vi "Cache_Hierarchy Global_Load All.vi"(8 "error in (no error)":errorcluster) -> (0 "error out":errorcluster, 1 "All Success?":bool, 3 "Hierarchy Map":map{string, string[]}(c390))   [LabVIEW 2019, in "ClassLoader.lvlib"]
doc: "Return paths to the ini cache files for all loaded PPLs."
uses:
  ClassLoader.lvlib
  Cache_Hierarchy Global.vi
  <vilib>/Utility/config.llb/NI_LVConfig.lvlib
  Ctl/Ctl_Hierarchy Cluster.ctl
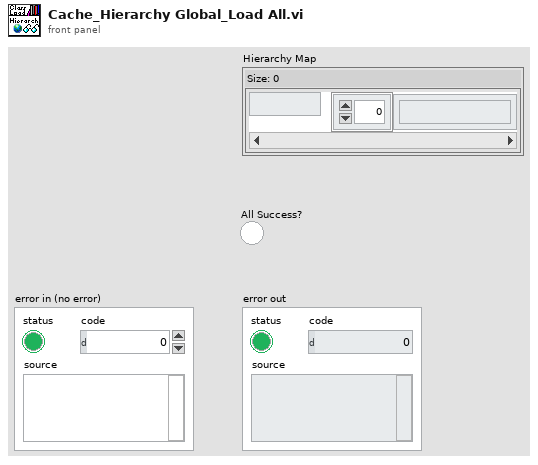
[diagram p1: front panel]
types:
  T1 = typedef "ClassLoader.lvlib/Ctl_Hierarchy Cluster.ctl" = cluster{"Hierarchy":string[]}
  T2 = typedef "NI_LVConfig.lvlib/Config Data RefNum.ctl" = refnum<k1>
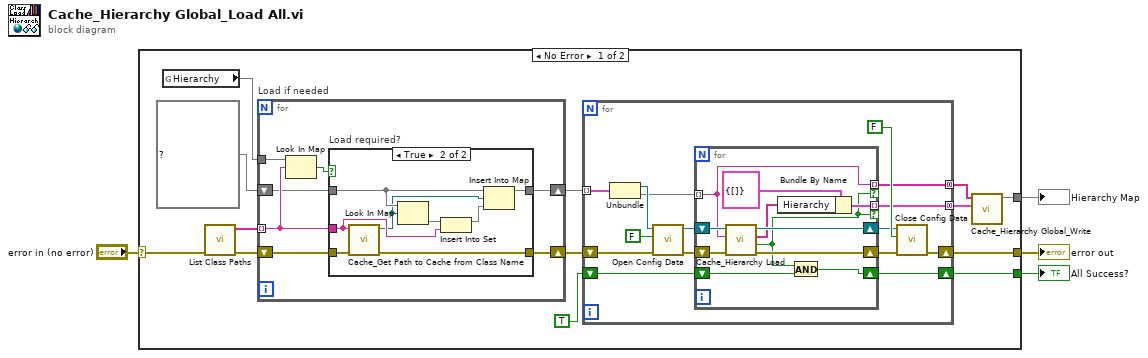
[diagram p0: block diagram]
diagram:
  n1 = case shown="No Error" "error in (no error)" {
    selector: "error in (no error)" -> [w17 w61]
    tunnel: [w10 w61] -> w3
    tunnel: [w7 _] -> w2
    tunnel: [w5 _] -> w1
    frame No Error {
      n2 = global read "Cache_Hierarchy Global.vi" "Hierarchy"() -> (w12:map{string, string[]})
      n3 = call "List Class Paths.vi"("error in (no error)"=w17) -> ("error out"=w13:errorcluster, "Class Names"=w16:string[])  [unwired: 8 in, 1 out]
      n4 = for "Load if needed" {
        tunnel: w16 -> [w48] mode=indexing
        tunnel: w12 -> [w49]
        shift-right: [w46] -> w11
        shift-left: map{path, set{string}} {} ("map") -> [w47]
        shift-right: [w45] -> w14
        shift-left: w13 -> [w44]
        n5 = Look In Map(map=w49, key=w48) -> (key not found?=w50:bool)  [unwired: 1 in, 1 out]
        n6 = case "Load required?" shown="True" w50 {
          tunnel: w48 -> [_ w59]
          tunnel: w47 -> [w52 w58]
          tunnel: [w52 w57] -> w46
          tunnel: [w51 w53] -> w45
          tunnel: w44 -> [w51 w54]
          frame False {
          }
          frame True {
            n7 = call "Cache_Get Path to Cache from Class Name.vi"("error in (no error)"=w54, "Class Name"=w59) -> ("error out"=w53:errorcluster, "Cache Path"=w56:path)  [unwired: 7 in, 1 out]
            n8 = Look In Map(map=w58, key=w56) -> (value=w60:set{string})  [unwired: 1 in, 1 out]
            n9 = Insert Into Set(10:w59, 11:w60) -> (3:w55:set{string})  [unwired: 1 out]
            n10 = Insert Into Map(map in=w58, key=w56, value=w55) -> (map out=w57:map{path, set{string}})  [unwired: 2 out]
          }
        }
      }
      n11 = for {
        tunnel: w11 -> [w32] mode=indexing
        shift-right: [w22] -> w10
        shift-left: w14 -> [w29]
        tunnel: [w21] -> w8 mode=concatenating
        tunnel: [w20] -> w9 mode=concatenating
        shift-right: [w18] -> w5
        shift-left: TRUE -> [w19]
        n12 = Unbundle(w32) -> ("Cache Path"=w30:path, "set"=w26:set{string})
        n13 = call <vilib>:"Open Config Data.vi"("error in (no error)"=w29, "create file if necessary (T)"=FALSE, "configuration file path"=w30) -> ("error out"=w24:errorcluster, "refnum"=w27:T2)  [unwired: 6 in, 1 out]
        n14 = for {
          shift-right: [w42] -> w25
          shift-left: w27 -> [w43]
          tunnel: w26 -> [w36] mode=indexing
          shift-right: [w40] -> w23
          shift-left: w24 -> [w41]
          tunnel: [w37] -> w21 mode=indexing if=w33
          tunnel: [w36] -> w20 mode=indexing if=w33
          shift-right: [w34] -> w18
          shift-left: w19 -> [w35]
          n15 = call "Cache_Hierarchy Load.vi"("error in (no error)"=w41, "Class Name"=w36, "Refnum in"=w43) -> ("error out"=w40:errorcluster, "Success?"=w33:bool, "Hierarchy"=w38:string[], "Refnum out"=w42:T2)  [unwired: 5 in]
          n16 = Bundle By Name(cluster=T1 {"Hierarchy"=[]} ("Hierarchy Cluster"), "Hierarchy"=w38) -> (w37:T1)
          n17 = And(x=w33, y=w35) -> (x .and. y?=w34:bool)
        }
        n18 = call <vilib>:"Close Config Data.vi"("error in (no error)"=w23, "write file if changed (T)"=FALSE, "refnum"=w25) -> ("error out"=w22:errorcluster)  [unwired: 7 in, 1 out]
      }
      n19 = call "Cache_Hierarchy Global_Write.vi"("Class Hierarchies"=w8, "Class Names"=w9) -> ("Hierarchy Map"=w7:map{string, string[]})  [unwired: 9 in]
    }
    frame Error {
    }
  }
  "error out" <- w3
  "Hierarchy Map" <- w2
  "All Success?" <- w1
